vi "Read Holding Registers.vi"(8 "error in":errorcluster, 9 "number of inputs":u16, 10 "starting address":u16, 11 "Modbus master in":refnum<class "Modbus Master.lvclass">) -> (0 "error out":errorcluster, 2 "register values":u16[](array[numeric]), 3 "Modbus master out":refnum<class "Modbus Master.lvclass">)   [LabVIEW 2014, in "MyLib.lvlib" / "Modbus Master.lvclass"]
doc: "Reads <B>number of inputs</B> holding registers starting at <B>starting address</B> from the device."
uses:
  Modbus Master.lvclass
  Modbus Master.lvclass/Modbus Master.ctl
  Modbus API.lvclass/Modbus API.ctl
  Transmission Data Unit/Transmission Data Unit.lvclass
  Modbus API.lvclass
  Master Function Definition/Master Function Definition.lvclass
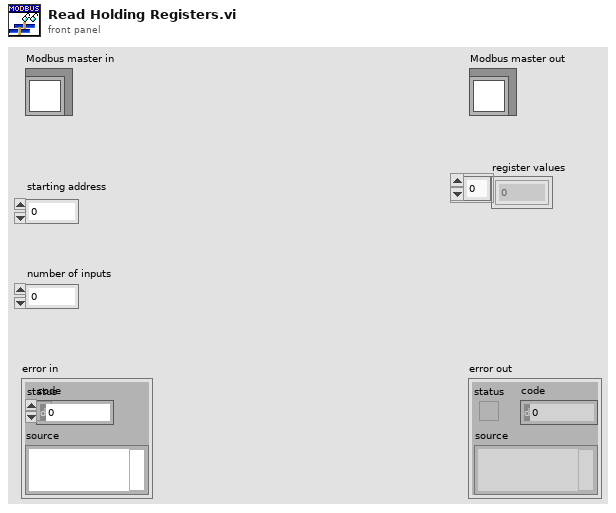
[diagram p1: front panel]
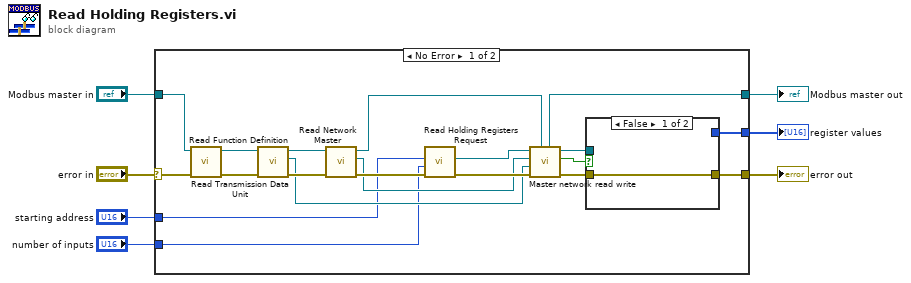
[diagram p0: block diagram]
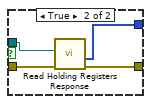
[diagram p2: hidden frame]
diagram:
  n1 = case shown="No Error" "error in" {
    selector: "error in" -> [w23 w33]
    tunnel: "number of inputs" -> [w12 _]
    tunnel: "starting address" -> [w13 _]
    tunnel: "Modbus master in" -> [w22 w34]
    tunnel: [w17 w34] -> w3
    tunnel: [w18 w33] -> w2
    tunnel: [w11 _] -> w1
    frame No Error {
      n2 = call "Read Function Definition.vi"("error in"=w23, "Modbus master in"=w22) -> ("error out"=w25:errorcluster, "Modbus master out"=w26:refnum<class "Modbus Master.lvclass">)  [unwired: 7 in, 1 out]
      n3 = call "Read Transmission Data Unit.vi"("error in"=w25, "Modbus instance in"=w26) -> ("error out"=w27:errorcluster, "transmission data unit"=w14:refnum<class "Transmission Data Unit.lvclass">, "Modbus instance out"=w24:refnum<class "Modbus Master.lvclass">)  [unwired: 7 in]
      n4 = call "Read Network Master.vi"("error in"=w27, "Modbus master in"=w24) -> ("error out"=w19:errorcluster, "network master"=w15:refnum<class "Network Master.lvclass">, "Modbus master out"=w16:refnum<class "Modbus Master.lvclass">)  [unwired: 7 in]
      n5 = call "Read Holding Registers Request.vi"("error in"=w19, "Number of Registers"=w12, "Starting Address"=w13) -> ("error out"=w20:errorcluster, "modbus data unit out"=w9:refnum<class "Modbus Data Unit.lvclass">)  [unwired: 7 in]
      n6 = call "Master network read write.vi"("Modbus master in"=w16, "error in"=w20, "transmission data unit in"=w14, "network master in"=w15, "Modbus data unit in"=w9) -> ("error out"=w21:errorcluster, "PDU Valid?"=w8:bool, "Modbus data unit out"=w10:refnum<class "Modbus Data Unit.lvclass">, "Modbus master out"=w17:refnum<class "Modbus Master.lvclass">)  [unwired: 3 in]
      n7 = case shown="False" w8 {
        tunnel: w21 -> [w28 w32]
        tunnel: [w28 w31] -> w18
        tunnel: [_ w30] -> w11
        tunnel: w10 -> [_ w29]
        frame False {
        }
        frame True {
          n8 = call "Read Holding Registers Response.vi"("error in"=w32, "modbus data unit in"=w29) -> ("error out"=w31:errorcluster, "Register Values"=w30:u16[])  [unwired: 7 in, 1 out]
        }
      }
    }
    frame Error {
    }
  }
  "Modbus master out" <- w3
  "error out" <- w2
  "register values" <- w1
